vi "ziAutoRange.vi"(8 "Error in":errorcluster, 10 "Path":string, 11 "Handle in":T1 {"Handle" format="0x%08x"; "Conn" format="0x%08x"}) -> (0 "Error out":errorcluster, 1 "Success":bool, 3 "Handle out":T1 {"Handle" format="0x%08x"; "Conn" format="0x%08x"})   [LabVIEW 2018, in "Zurich Instruments LabOne.lvlib"]
doc: "Automatically set the input range of signalinputs/{0,1} to half full level.\n<B>Path</B> can either be sigins/0 or sigins/1"
uses:
  Zurich Instruments LabOne.lvlib
  <vilib>/regexp/Match Regular Expression.xnode
  Configure/ziGetValueString.vi
  ziTypeHandle.ctl
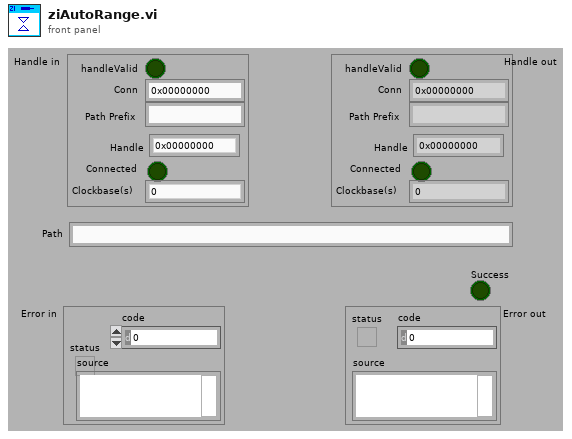
[diagram p1: front panel]
types:
  T1 = typedef "Zurich Instruments LabOne.lvlib/ziTypeHandle.ctl" = cluster{"handleValid":bool, "Conn":u64, "Path Prefix":string, "Handle":u64, "Connected":bool, "Clockbase(s)":dbl}
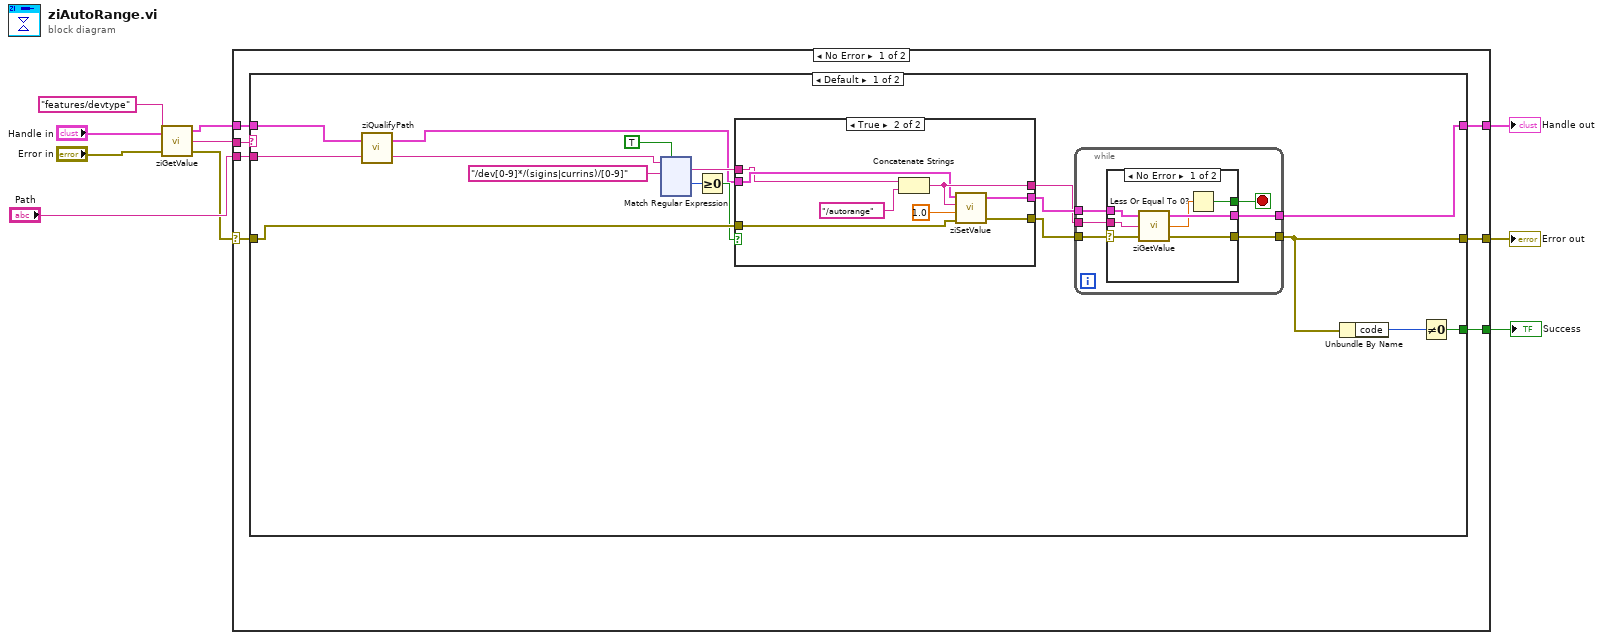
[diagram p0: block diagram]
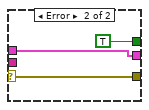
[diagram p2: hidden frame]
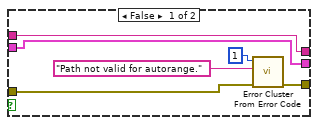
[diagram p3: hidden frame]
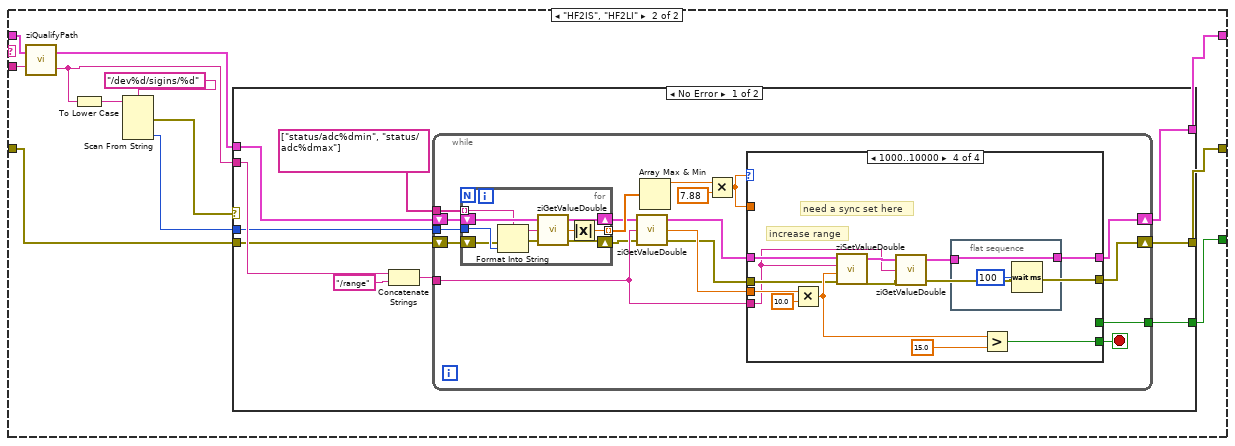
[diagram p4: hidden frame]
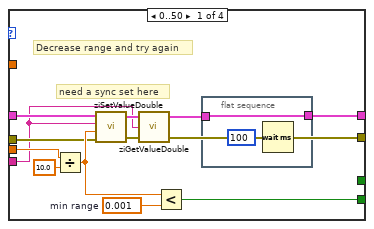
[diagram p5: hidden frame]
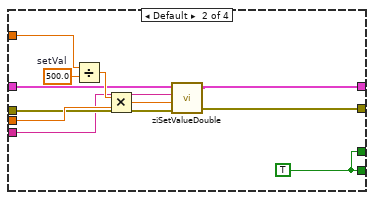
[diagram p6: hidden frame]
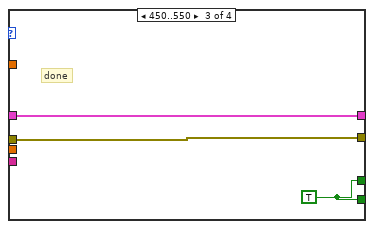
[diagram p7: hidden frame]
diagram:
  n1 = call-poly "ziGetValue.vi"("error in"="Error in", "Path"="features/devtype", "Handle In"="Handle in") -> ("error out"=w2:errorcluster, "Value"=w1:string, "Handle Out"=w3:T1)
  n2 = case shown="No Error" w2 {
    selector: w2 -> [w15 w268]
    tunnel: [w17 w268] -> w10
    tunnel: [w16 w269] -> w9
    tunnel: w3 -> [w13 w269]
    tunnel: "Path" -> [w14 _]
    tunnel: [w12 _] -> w7
    tunnel: w1 -> [w11 _]
    frame No Error {
      n3 = case shown="Default" w11 {
        tunnel: [w25 w183] -> w17
        tunnel: [w32 w182] -> w16
        tunnel: w15 -> [w34 w181]
        tunnel: w14 -> [w22 w180]
        tunnel: w13 -> [w23 w179]
        tunnel: [w19 w175] -> w12
        frame Default {
          n4 = call "ziQualifyPath.vi"("Path In"=w22, "Handle In"=w23) -> ("Path Out"=w18:string, "Handle Out"=w21:T1)
          n5 = xnode "Match Regular Expression"("input string"=w18, "regular expression"="/dev[0-9]*/(sigins|currins)/[0-9]", "ignore case? (F)"=TRUE) -> ("whole match"=w29:string, "offset past match"=w27:i32)  [unwired: 3 in, 3 out]
          n6 = Greater Or Equal To 0?(x=w27) -> (x >= 0?=w28:bool)
          n7 = case shown="True" w28 {
            tunnel: w34 -> [w161 w171]
            tunnel: w21 -> [w163 w165]
            tunnel: [w163 w168] -> w33
            tunnel: [w162 w167] -> w31
            tunnel: [w160 w166] -> w30
            tunnel: w29 -> [w162 w164]
            frame False {
              n8 = call <vilib>:"Error Cluster From Error Code.vi"("error in (no error)"=w161, "error message (\"\")"="Path not valid for autorange." ("error message (\"\")"), "error code (0)"=1) -> ("error out"=w160:errorcluster)  [unwired: 6 in]
            }
            frame True {
              n9 = Concatenate Strings(w164, "/autorange") -> (w167:string)
              n10 = call-poly "ziSetValue.vi"("Error In"=w171, "Value"=1.0, "Path"=w167, "Handle In"=w165) -> ("Error Out"=w166:errorcluster, "Handle Out"=w168:T1)  [unwired: 1 in]
            }
          }
          n11 = while {
            tunnel: w30 -> [w35]
            tunnel: w33 -> [w40]
            tunnel: [w39] -> w32
            tunnel: w31 -> [w38]
            tunnel: [w36] -> w25
            stop <- w37 stop-if-true
            n12 = case shown="No Error" w35 {
              selector: w35 -> [w41 w49]
              tunnel: w40 -> [w47 w50]
              tunnel: [w46 w50] -> w39
              tunnel: w38 -> [w45 _]
              tunnel: [w44 TRUE] -> w37
              tunnel: [w42 w49] -> w36
              frame No Error {
                n13 = call-poly "ziGetValue.vi"("error in"=w41, "Path"=w45, "Handle in"=w47) -> ("error out"=w42:errorcluster, "Value"=w43:dbl, "Handle out"=w46:T1)
                n14 = Less Or Equal To 0?(x=w43) -> (x <= 0?=w44:bool)
              }
              frame Error {
              }
            }
          }
          n15 = Unbundle By Name(w25) -> ("code"=w20:i32)
          n16 = Not Equal To 0?(x=w20) -> (x != 0?=w19:bool)
        }
        frame "HF2IS", "HF2LI" {
          n17 = call "ziQualifyPath.vi"("Path In"=w180, "Handle In"=w179) -> ("Path Out"=w174:string, "Handle Out"=w178:T1)
          n18 = To Lower Case(string=w174) -> (all lower case string=w173:string)
          n19 = Scan From String(format string="/dev%d/sigins/%d" ("regular expression"), input string=w173) -> (error out=w177:errorcluster, output 2=w172:i32)  [unwired: 5 in, 2 out]
          n20 = case shown="No Error" w177 {
            tunnel: [w190 w267] -> w183
            tunnel: [w191 w266] -> w182
            tunnel: w178 -> [w192 w266]
            tunnel: w181 -> [w184 w267]
            tunnel: w174 -> [w187 _]
            tunnel: w172 -> [w185 _]
            tunnel: [w186 _] -> w175
            frame No Error {
              n21 = Concatenate Strings(w187, "/range") -> (w189:string)
              n22 = while {
                shift-right: [w208] -> w191
                shift-left: w192 -> [w204]
                shift-right: [w207] -> w190
                shift-left: w184 -> [w196]
                tunnel: w189 -> [w199]
                tunnel: string[] ["status/adc%dmin", "status/adc%dmax"] -> [w203]
                tunnel: w185 -> [w195]
                tunnel: [w194] -> w186
                stop <- w206 stop-if-true
                n23 = for {
                  tunnel: w203 -> [w216] mode=indexing
                  tunnel: [w221] -> w211 mode=indexing
                  shift-right: [w220] -> w202
                  shift-left: w204 -> [w219]
                  tunnel: w195 -> [w215]
                  shift-right: [w217] -> w197
                  shift-left: w196 -> [w213]
                  n24 = Format Into String(format string=w216, error in=w213, w215) -> (resulting string=w214:string, error out=w212:errorcluster)  [unwired: 1 in]
                  n25 = call "ziGetValueDouble.vi"("error in"=w212, "Path"=w214, "Handle in"=w219) -> ("error out"=w217:errorcluster, "Value"=w218:dbl, "Handle out"=w220:T1)
                  n26 = Absolute Value(x=w218) -> (abs(x)=w221:dbl)
                }
                n27 = call "ziGetValueDouble.vi"("error in"=w197, "Path"=w199, "Handle in"=w202) -> ("error out"=w198:errorcluster, "Value"=w200:dbl, "Handle out"=w201:T1)
                n28 = Array Max & Min(array=w211) -> (max value=w209:dbl)  [unwired: 3 out]
                n29 = Multiply(x=w209, y=7.88 ("valueD")) -> (x*y=w205:dbl)
                n30 = case shown="1000..10000" w205 {
                  tunnel: w201 -> [w231 w241 w249 w259]
                  tunnel: w198 -> [w229 w239 w250 w257]
                  tunnel: [w224 w243 w249 w253] -> w208
                  tunnel: [w223 w242 w250 w252] -> w207
                  tunnel: [w222 w237 w248 w260] -> w206
                  tunnel: w200 -> [w234 w247 _ w262]
                  tunnel: w205 -> [_ w245 _ _]
                  tunnel: w199 -> [w227 w238 _ w251]
                  tunnel: [_ w237 w248 _] -> w194
                  frame 0..50 {
                    w232 = 0.001  # min range
                    # "need a sync set here"
                    # "Decrease range and try again"
                    n31 = Divide(x=w234, y=10.0 ("valueD")) -> (x/y=w230:dbl)
                    n32 = call "ziSetValueDouble.vi"("Error In"=w229, "Value"=w230, "Path"=w227, "Handle In"=w231) -> ("Error Out"=w226:errorcluster, "Handle Out"=w228:T1)  [unwired: 1 in]
                    n33 = call "ziGetValueDouble.vi"("error in"=w226, "Path"=w227, "Handle in"=w228) -> ("error out"=w223:errorcluster, "Handle out"=w225:T1)  [unwired: 1 out]
                    n34 = Less?(x=w230, y=w232) -> (x < y?=w222:bool)
                    n35 = flat-sequence {
                      tunnel: w225 -> [w235]
                      tunnel: [w235] -> w224
                      frame #0 {
                        n36 = Wait (ms)(milliseconds to wait=u32 100) -> ()  [unwired: 1 out]
                      }
                    }
                  }
                  frame Default {
                    w244 = 500.0  # setVal
                    w237 = TRUE
                    n37 = Divide(x=w245, y=w244) -> (x/y=w246:dbl)
                    n38 = Multiply(x=w246, y=w247) -> (x*y=w240:dbl)
                    n39 = call "ziSetValueDouble.vi"("Error In"=w239, "Value"=w240, "Path"=w238, "Handle In"=w241) -> ("Error Out"=w242:errorcluster, "Handle Out"=w243:T1)  [unwired: 1 in]
                  }
                  frame 450..550 {
                    w248 = TRUE
                    # "done"
                  }
                  frame 1000..10000 {
                    # "need a sync set here"
                    # "increase range"
                    n40 = Multiply(x=w262, y=10.0 ("valueD")) -> (x*y=w258:dbl)
                    n41 = call "ziSetValueDouble.vi"("Error In"=w257, "Value"=w258, "Path"=w251, "Handle In"=w259) -> ("Error Out"=w255:errorcluster, "Handle Out"=w256:T1)  [unwired: 1 in]
                    n42 = call "ziGetValueDouble.vi"("error in"=w255, "Path"=w251, "Handle in"=w256) -> ("error out"=w252:errorcluster, "Handle out"=w254:T1)  [unwired: 1 out]
                    n43 = flat-sequence {
                      tunnel: w254 -> [w264]
                      tunnel: [w264] -> w253
                      frame #0 {
                        n44 = Wait (ms)(milliseconds to wait=u32 100) -> ()  [unwired: 1 out]
                      }
                    }
                    n45 = Greater?(x=w258, y=15.0 ("valueD")) -> (0:w260:bool)
                  }
                }
              }
            }
            frame Error {
            }
          }
        }
      }
    }
    frame Error {
    }
  }
  "Handle out" <- w9
  "Error out" <- w10
  "Success" <- w7
